vi "Event Handler_Pretzel Dispenser.vi"() -> ()   [LabVIEW 2020]
panel:
  out "Money\nInserted ($)":dbl format="%.2g"
  out "$ Charged":dbl
  out "Change\nDispensed ($)":dbl format="%.2f"
  out "Dispense\nChange":bool
  out "Vend":bool
  in  "Payment\nType":T1(ring)
  in  "Insert Payment":bool
  in  "Initialize":bool
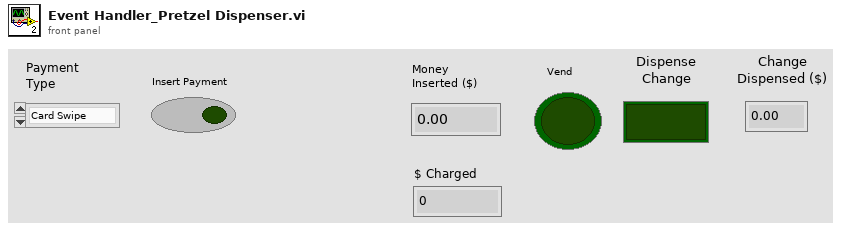
[diagram p1: front panel]
types:
  T1 = enum16{"Card Swipe", "Nickel", "Dime", "Quarter", "Shutdown", "Vend", "Change", "Wait", "Initialize"}
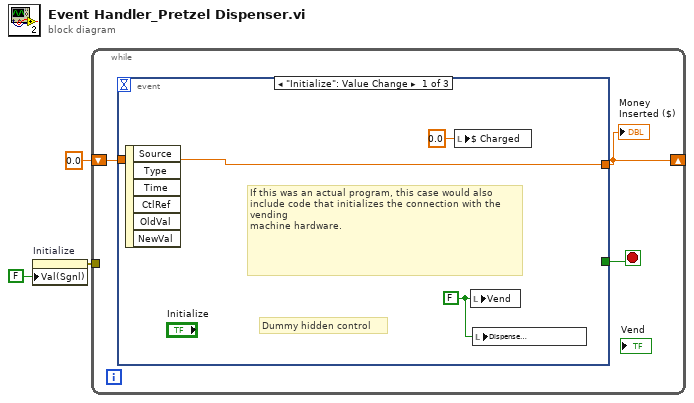
[diagram p0: block diagram]
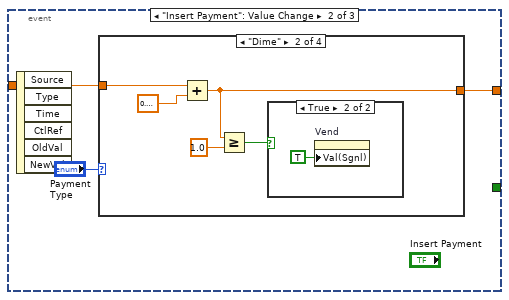
[diagram p2: hidden frame]
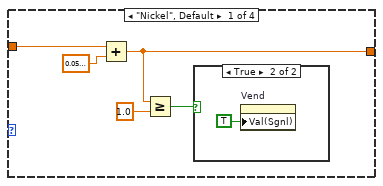
[diagram p3: hidden frame]
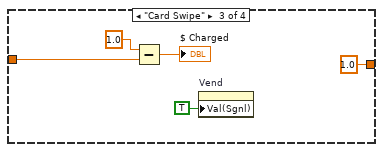
[diagram p6: hidden frame]
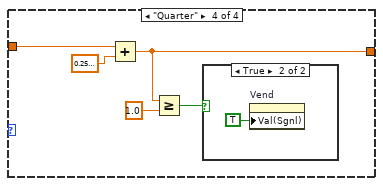
[diagram p7: hidden frame]
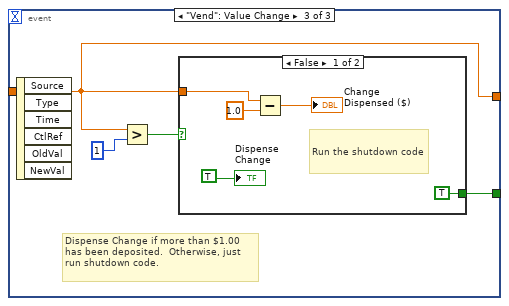
[diagram p9: hidden frame]
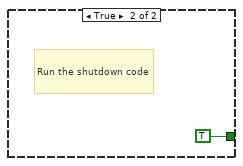
[diagram p10: hidden frame]
diagram:
  n1 = property on="Initialize" class="Bool (strict)"("Val(Sgnl)"=FALSE ("Value (Signaling)")) -> (error out=w2:errorcluster)  [unwired: 2 in, 1 out]
  n2 = while {
    tunnel: w2 -> [_]
    shift-right: [w5] -> _
    shift-left: 0.0 -> [w6]
    stop <- w4 stop-if-true
    n3 = event shown="[0] \"Initialize\": Value Change" {
      selector: _ -> [_ _ _]
      dyn-events: _ -> [_ _ _]
      timeout: _ -> [_ _ _]
      tunnel: w6 -> [w9 w11 w37]
      tunnel: [w9 w10 w37] -> w5
      tunnel: [_ _ w36] -> w4
      event "Initialize": Value Change {
        w8 = FALSE ("Vend")
        # "Dummy hidden control"
        # "If this was an actual program, this case would also include code that initializes the connection with the vending\nmachine hardware."
        n4 = event-data() -> ()  [unwired: 1 in, 6 out]
        n5 = local write "$ Charged"(0.0 ("$ Charged")) -> ()
        n6 = local write "Vend"(w8) -> ()
        n7 = local write "Dispense\nChange"(w8) -> ()
      }
      event "Insert Payment": Value Change {
        n8 = event-data() -> ()  [unwired: 1 in, 6 out]
        n9 = case shown="\"Dime\"" "Payment\nType" {
          tunnel: w11 -> [w14 w23 w27 w34]
          tunnel: [w13 w19 1.0 w30] -> w10
          frame "Nickel", Default {
            n10 = Add(x=w14, y=0.0500000001) -> (x+y=w13:dbl)
            n11 = Greater Or Equal?(x=w13, y=1.0) -> (x >= y?=w17:bool)
            n12 = case shown="True" w17 {
              frame False {
              }
              frame True {
                n13 = property on="Vend" class="Bool (strict)"("Val(Sgnl)"=TRUE ("Value (Signaling)")) -> ()  [unwired: 2 in, 2 out]
              }
            }
          }
          frame "Dime" {
            n14 = Add(x=w23, y=0.10000000149011612) -> (x+y=w19:dbl)
            n15 = Greater Or Equal?(x=w19, y=1.0) -> (x >= y?=w21:bool)
            n16 = case shown="True" w21 {
              frame False {
              }
              frame True {
                n17 = property on="Vend" class="Bool (strict)"("Val(Sgnl)"=TRUE ("Value (Signaling)")) -> ()  [unwired: 2 in, 2 out]
              }
            }
          }
          frame "Card Swipe" {
            n18 = Subtract(x=1.0, y=w27) -> (x-y=→"$ Charged":dbl)
            n19 = property on="Vend" class="Bool (strict)"("Val(Sgnl)"=TRUE ("Value (Signaling)")) -> ()  [unwired: 2 in, 2 out]
          }
          frame "Quarter" {
            n20 = Add(x=w34, y=0.2500000001) -> (x+y=w30:dbl)
            n21 = Greater Or Equal?(x=w30, y=1.0) -> (x >= y?=w32:bool)
            n22 = case shown="True" w32 {
              frame False {
              }
              frame True {
                n23 = property on="Vend" class="Bool (strict)"("Val(Sgnl)"=TRUE ("Value (Signaling)")) -> ()  [unwired: 2 in, 2 out]
              }
            }
          }
        }
      }
      event "Vend": Value Change {
        # "Dispense Change if more than $1.00 has been deposited.  Otherwise, just run shutdown code."
        n24 = event-data() -> ()  [unwired: 1 in, 6 out]
        n25 = Greater?(x=w37, y=1) -> (0:w38:bool)
        n26 = case shown="False" w38 {
          tunnel: w37 -> [w42 _]
          tunnel: [TRUE TRUE] -> w36
          frame False {
            # "Run the shutdown code"
            n27 = Subtract(x=w42, y=1.0) -> (x-y=→"Change\nDispensed ($)":dbl)
            "Dispense\nChange" <- TRUE ("Dispense\nChange")
          }
          frame True {
            # "Run the shutdown code"
          }
        }
      }
    }
    "Money\nInserted ($)" <- w5
  }
